vi "Pumps_Valves_Dependencies_Global.vi"() -> ()   [LabVIEW 2011]
panel:
  in  "Density Required (kg/m3)":dbl
  out "V30,V28":bool
  in  "Towing Tank":dbl
  in  "Tank D":dbl
  in  "Tank C":dbl
  in  "Tank B":dbl
  in  "Tank A":dbl
  in  "Salt Saturator":dbl
  out "V9,V15,V33":bool
  in  "Tanks":dbl[](array[numeric])
  out "V29,V28":bool
  out "M.P, V.P":bool
  out "M.P, P.P":bool
  in  "V14,V31":bool
  in  "V12,V31":bool
  in  "V6,V31":bool
  in  "V9,V13,V19":bool
  in  "V7,V19/V18":bool
  in  "V5,V33,V19":bool
  in  "V4,V33,V19":bool
  in  "V29,V23":bool
  in  "V29,V27":bool
  in  "Pump D":bool
  in  "Pump C":bool
  in  "Pump B":bool
  in  "Pump A":bool
  in  "Valve Power":bool
  in  "Pump Power":bool
  in  "Main Rack Power":bool
  in  "V34":bool
  in  "V33":bool
  in  "V32":bool
  in  "V31":bool
  in  "V30":bool
  in  "V29":bool
  in  "V28":bool
  in  "V27":bool
  in  "V26":bool
  in  "V25":bool
  in  "V24":bool
  in  "V23":bool
  in  "V22":bool
  in  "V21":bool
  in  "V20":bool
  in  "V19":bool
  in  "V18":bool
  in  "V15":bool
  in  "V14":bool
  in  "V13":bool
  in  "V12":bool
  in  "V11":bool
  in  "V10":bool
  in  "V9":bool
  in  "V8":bool
  in  "V7":bool
  in  "V6":bool
  in  "V5":bool
  in  "V4":bool
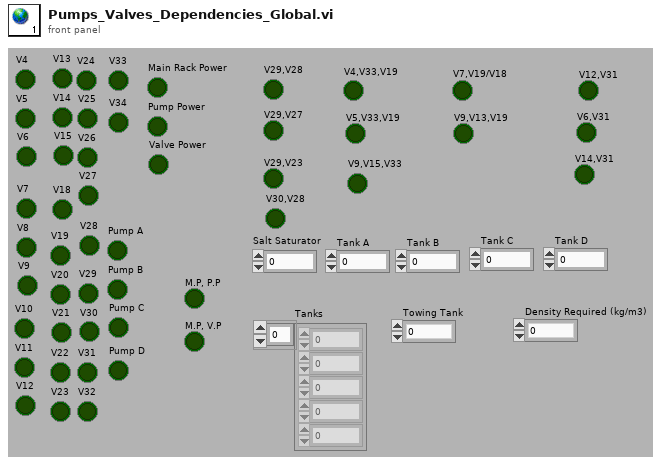
[diagram p1: front panel]
diagram:
